vi "Client - Main.vi"() -> ()   [LabVIEW 2020]
uses:
  shared/controls/Ports to Check.ctl
  shared/controls/Client States.ctl
panel:
  out "Message from Server":string
  out "Connection Established?":bool
  in  "InsightCM Server Address":string="127.0.0.1"
  in  "User Panel":enum32{"User Panel"}(tab)
  in  "stop":bool
  in  "Establish Connection":bool
  in  "Start Test":bool
  in  "View Results":bool
  in  "Log Results":bool
  out "error out":errorcluster
  out "Ports to Check":T1={"TCP Ports"=[82, 482, 5672, 6343, 8002, 49580, 3580, 80, 22, 44516, 52725, 8080], "UDP Ports"=[5353, 44515, 44525]}
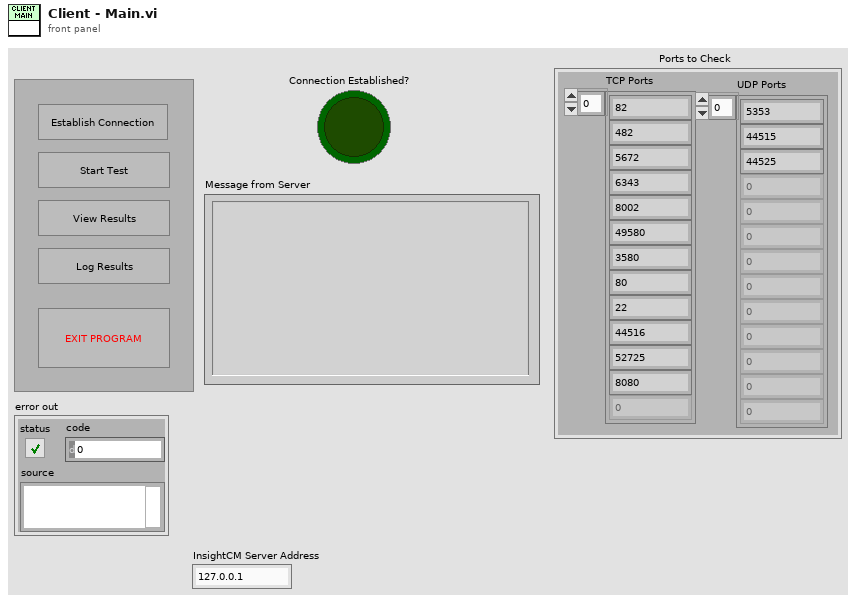
[diagram p1: front panel]
types:
  T1 = typedef "Ports to Check.ctl" = cluster{"TCP Ports":u32[], "UDP Ports":u32[]}
  T2 = typedef "Client States.ctl" = enum16{"Initialize", "Idle", "Establish Connection", "Start Test", "TCP Tests", "UDP Tests", "Test Complete", "View Results", "Log Results", "Edit Configuration", "Stop"}
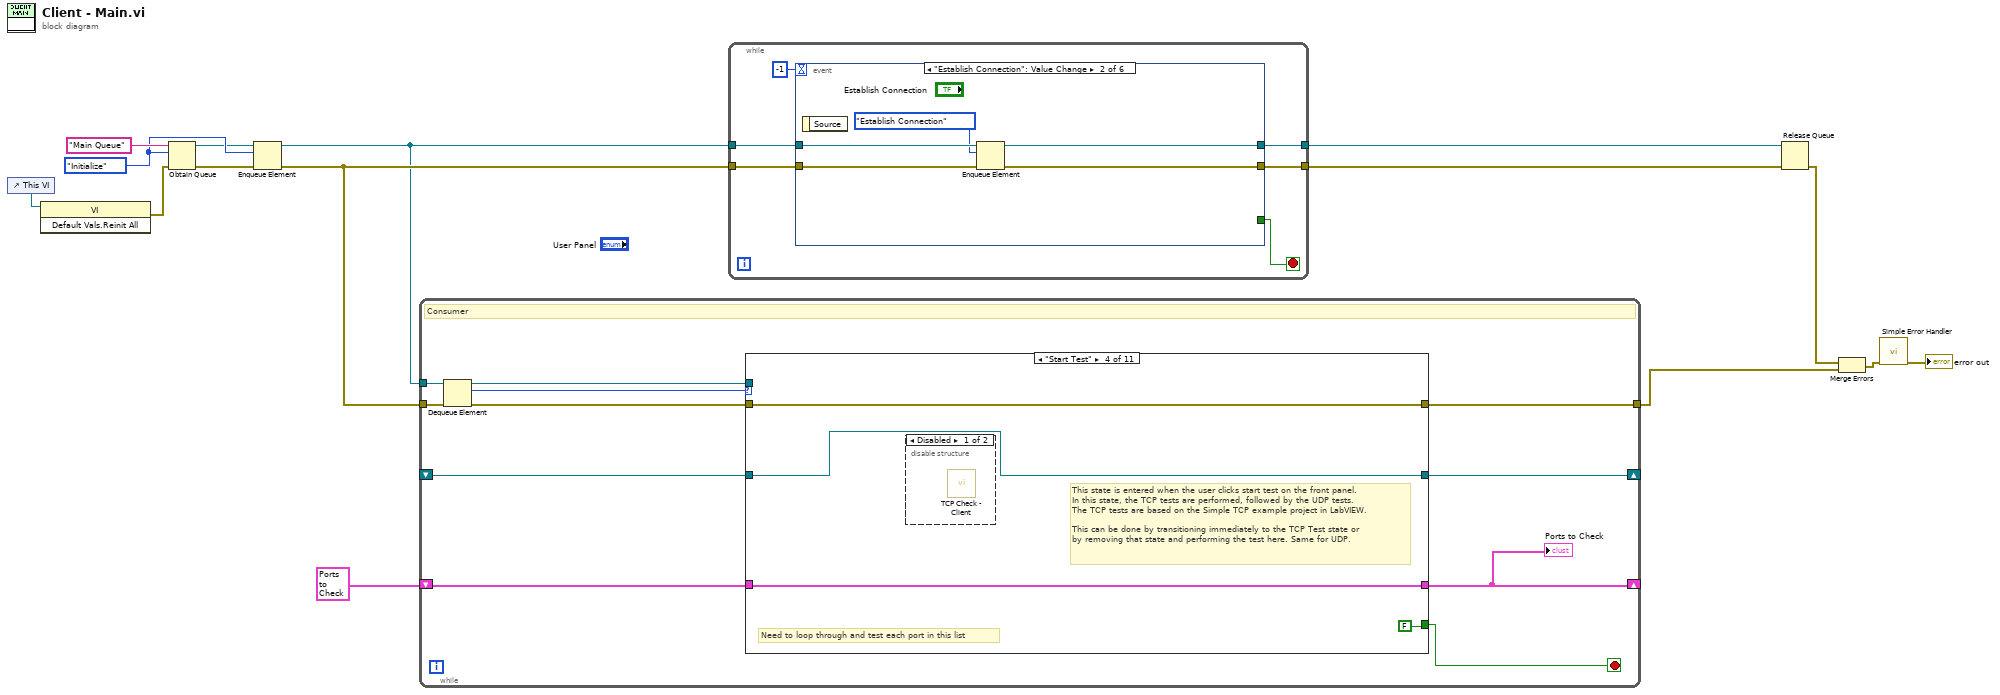
[diagram p0: block diagram]
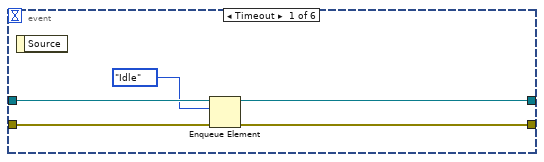
[diagram p2: hidden frame]
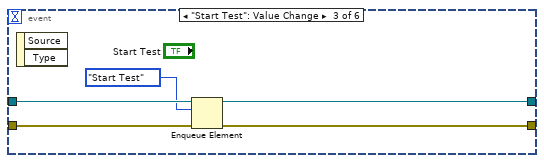
[diagram p3: hidden frame]
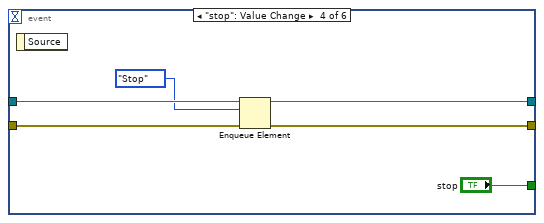
[diagram p4: hidden frame]
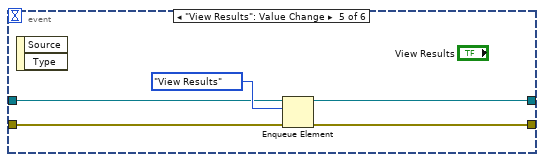
[diagram p5: hidden frame]
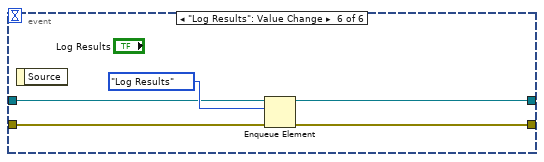
[diagram p6: hidden frame]
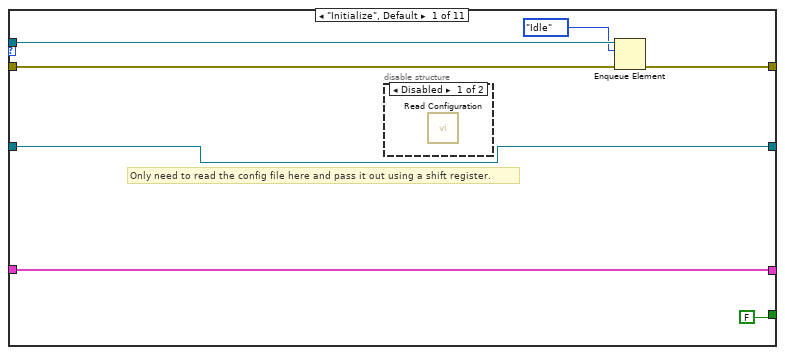
[diagram p7: hidden frame]
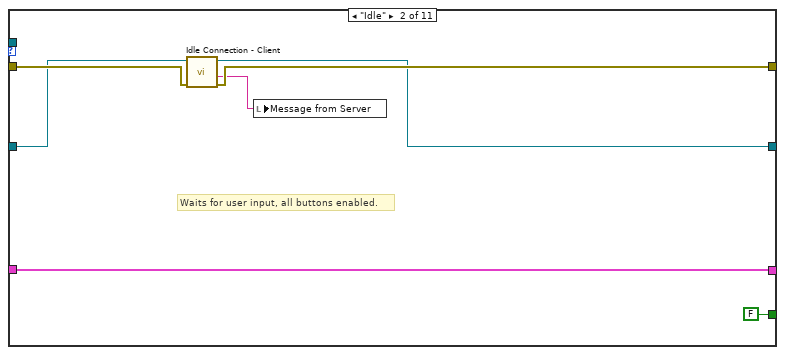
[diagram p9: hidden frame]
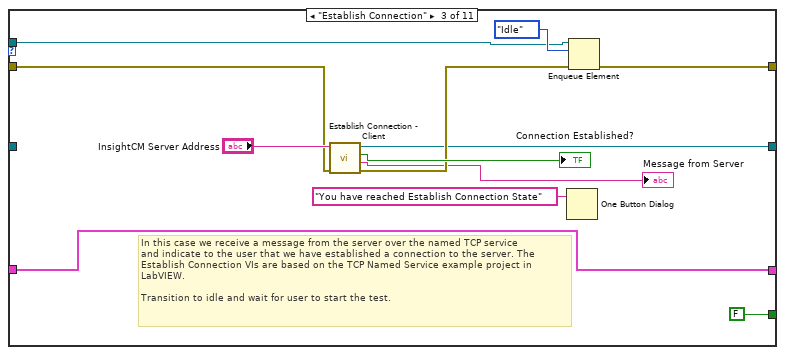
[diagram p10: hidden frame]
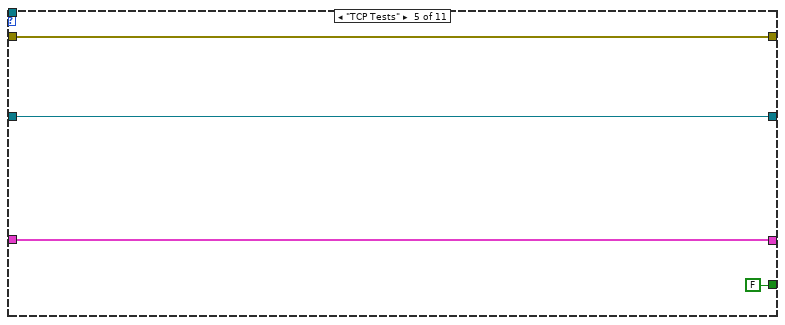
[diagram p12: hidden frame]
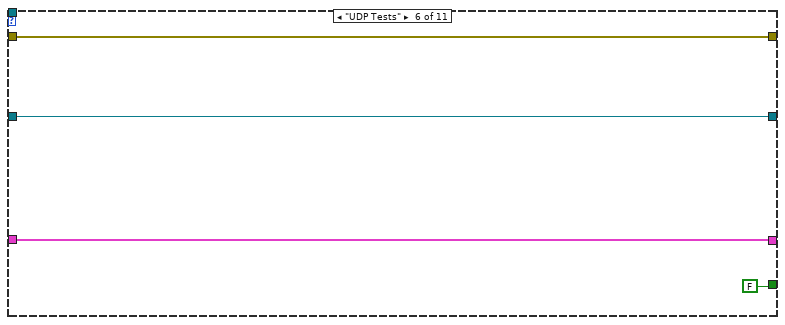
[diagram p13: hidden frame]
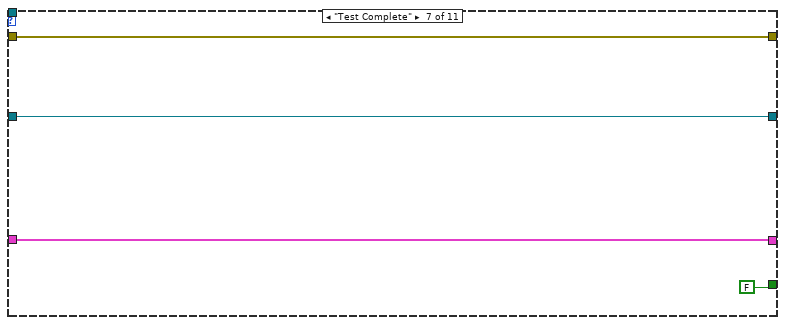
[diagram p14: hidden frame]
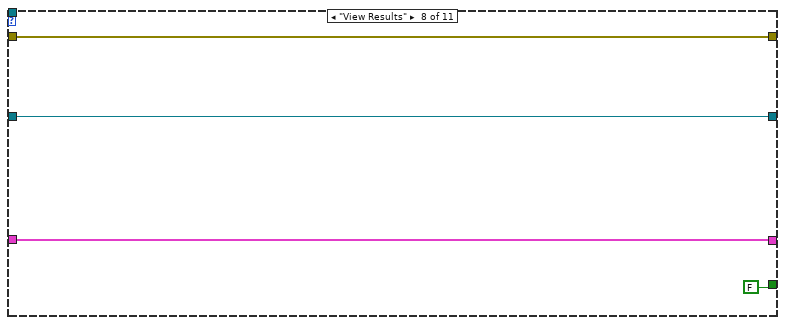
[diagram p15: hidden frame]
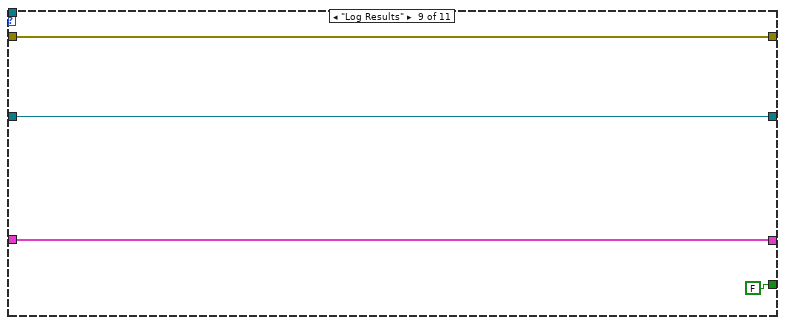
[diagram p16: hidden frame]
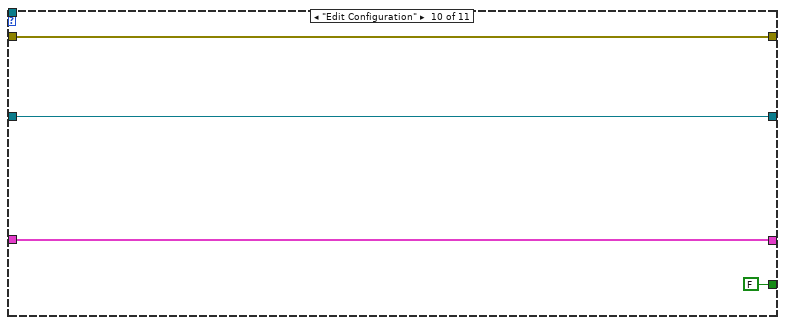
[diagram p17: hidden frame]
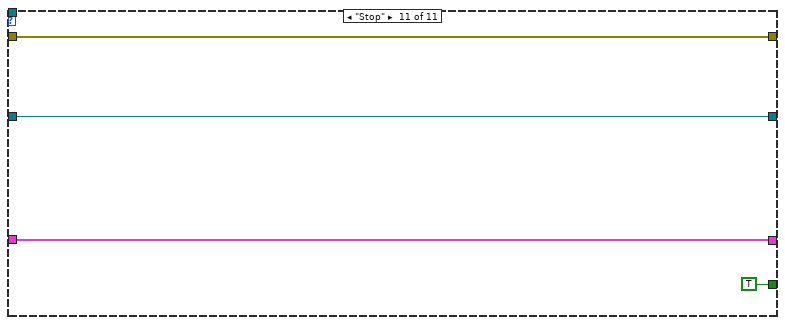
[diagram p18: hidden frame]
diagram:
  w5 = Client_States."Initialize" ("States")
  n1 = control-ref of="This VI"() -> (w8:refnum<vi>)
  n2 = invoke class="VI" method="Default Vals.Reinit All"(reference=w8) -> (error out=w7:errorcluster)  [unwired: 2 in, 2 out]
  n3 = Obtain Queue(name (unnamed)="Main Queue", element data type=w5, error in (no error)=w7) -> (queue out=w3:refnum<queue>, error out=w9:errorcluster)  [unwired: 2 in, 1 out]
  n4 = Enqueue Element(queue=w3, element=w5, error in (no error)=w9) -> (queue out=w4:refnum<queue>, error out=w6:errorcluster)  [unwired: 1 in, 1 out]
  n5 = while {
    tunnel: w4 -> [w26]
    tunnel: w6 -> [w25]
    shift-right: [w22] -> _
    shift-left: T1 {"TCP Ports"=[82, 482, 5672, 6343, 8002, 49580, 3580, 80, 22, 44516, 52725, 8080], "UDP Ports"=[5353, 44515, 44525]} ("Ports to Check") -> [w21]
    tunnel: [w19] -> w1
    shift-right: [w17] -> _
    shift-left: _ -> [w16]
    stop <- w18 stop-if-true
    # "Consumer"
    n6 = Dequeue Element(queue=w26, error in (no error)=w25) -> (queue out=w23:refnum<queue>, element=w24:T2, error out=w20:errorcluster)  [unwired: 1 in, 1 out]
    n7 = case shown="\"Start Test\"" w24 {
      tunnel: w23 -> [w33 _ w49 _ _ _ _ _ _ _ _]
      tunnel: [w30 w40 w51 w56 w60 w64 w68 w72 w76 w80 w84] -> w22
      tunnel: w21 -> [w30 w40 w51 w56 w60 w64 w68 w72 w76 w80 w84]
      tunnel: w20 -> [w31 w38 w46 w55 w59 w63 w67 w71 w75 w79 w83]
      tunnel: [w28 w36 w48 w55 w59 w63 w67 w71 w75 w79 w83] -> w19
      tunnel: [FALSE FALSE FALSE FALSE FALSE FALSE FALSE FALSE FALSE FALSE TRUE] -> w18
      tunnel: [w27 w35 w41 w53 w57 w61 w65 w69 w73 w77 w81] -> w17
      tunnel: w16 -> [w27 w37 _ w53 w57 w61 w65 w69 w73 w77 w81]
      frame "Initialize", Default {
        # "Only need to read the config file here and pass it out using a shift register."
        n8 = disable-structure shown="Disabled" {
          frame Disabled {
            n9 = call "Read Configuration.vi"() -> ()  [unwired: 10 in, 2 out]
          }
          frame Enabled {
          }
        }
        n10 = Enqueue Element(queue=w33, element=Client_States."Idle" ("States"), error in (no error)=w31) -> (error out=w28:errorcluster)  [unwired: 1 in, 2 out]
      }
      frame "Idle" {
        # "Waits for user input, all buttons enabled."
        n11 = call "Idle Connection - Client.vi"("connection ID"=w37, "error in (no error)"=w38) -> ("connection ID out"=w35:refnum<k5>, "Message from Server"=w34:string, "No error"=w36:errorcluster)  [unwired: 5 in, 1 out]
        n12 = local write "Message from Server"(w34) -> ()
      }
      frame "Establish Connection" {
        # "In this case we receive a message from the server over the named TCP service \nand indicate to the user that we have established a connection to the server. The \nEstablish Connection VIs are based on the TCP Named Service example project in \nLabVIEW. \n\nTransition to idle and wait for user to start the test."
        n13 = call "Establish Connection - Client.vi"("server address"="InsightCM Server Address", "error in (no error)"=w46) -> ("connection ID out"=w41:refnum<k5>, "Connection Established?"=→"Connection Established?":bool, "Message from Server"=→"Message from Server":string, "No error"=w45:errorcluster)  [unwired: 5 in]
        n14 = One Button Dialog(message="You have reached Establish Connection State") -> ()  [unwired: 1 in, 1 out]
        n15 = Enqueue Element(queue=w49, element=Client_States."Idle" ("States"), error in (no error)=w45) -> (error out=w48:errorcluster)  [unwired: 1 in, 2 out]
      }
      frame "Start Test" {
        # "Need to loop through and test each port in this list"
        # "This state is entered when the user clicks start test on the front panel.\nIn this state, the TCP tests are performed, followed by the UDP tests.\nThe TCP tests are based on the Simple TCP example project in LabVIEW.\n\nThis can be done by transitioning immediately to the TCP Test state or \nby removing that state and performing the test here. Same for UDP."
        n16 = disable-structure shown="Disabled" {
          frame Disabled {
            n17 = call "TCP Check - Client.vi"() -> ()  [unwired: 8 in, 3 out]
          }
          frame Enabled {
          }
        }
      }
      frame "TCP Tests" {
      }
      frame "UDP Tests" {
      }
      frame "Test Complete" {
      }
      frame "View Results" {
      }
      frame "Log Results" {
      }
      frame "Edit Configuration" {
      }
      frame "Stop" {
      }
    }
    "Ports to Check" <- w22
  }
  n18 = while {
    tunnel: w4 -> [w90]
    tunnel: [w89] -> w14
    tunnel: w6 -> [w87]
    tunnel: [w86] -> w11
    stop <- w88 stop-if-true
    n19 = event shown="[1] \"Establish Connection\": Value Change" {
      selector: _ -> [_ _ _ _ _ _]
      dyn-events: _ -> [_ _ _ _ _ _]
      timeout: -1 -> [_ _ _ _ _ _]
      tunnel: w90 -> [w95 w100 w105 w110 w115 w120]
      tunnel: [w94 w98 w103 w109 w114 w119] -> w89
      tunnel: [_ _ _ "stop" _ _] -> w88
      tunnel: w87 -> [w93 w97 w102 w107 w113 w118]
      tunnel: [w92 w96 w101 w106 w112 w117] -> w86
      event Timeout {
        n20 = event-data() -> ()  [unwired: 1 in, 1 out]
        n21 = Enqueue Element(queue=w95, element=Client_States."Idle" ("States"), error in (no error)=w93) -> (queue out=w94:refnum<queue>, error out=w92:errorcluster)  [unwired: 1 in, 1 out]
      }
      event "Establish Connection": Value Change {
        n22 = event-data() -> ()  [unwired: 1 in, 1 out]
        n23 = Enqueue Element(queue=w100, element=Client_States."Establish Connection" ("States"), error in (no error)=w97) -> (queue out=w98:refnum<queue>, error out=w96:errorcluster)  [unwired: 1 in, 1 out]
      }
      event "Start Test": Value Change {
        n24 = event-data() -> ()  [unwired: 1 in, 2 out]
        n25 = Enqueue Element(queue=w105, element=Client_States."Start Test" ("States"), error in (no error)=w102) -> (queue out=w103:refnum<queue>, error out=w101:errorcluster)  [unwired: 1 in, 1 out]
      }
      event "stop": Value Change {
        n26 = event-data() -> ()  [unwired: 1 in, 1 out]
        n27 = Enqueue Element(queue=w110, element=Client_States."Stop" ("States"), error in (no error)=w107) -> (queue out=w109:refnum<queue>, error out=w106:errorcluster)  [unwired: 1 in, 1 out]
      }
      event "View Results": Value Change {
        n28 = event-data() -> ()  [unwired: 1 in, 2 out]
        n29 = Enqueue Element(queue=w115, element=Client_States."View Results" ("States"), error in (no error)=w113) -> (queue out=w114:refnum<queue>, error out=w112:errorcluster)  [unwired: 1 in, 1 out]
      }
      event "Log Results": Value Change {
        n30 = event-data() -> ()  [unwired: 1 in, 1 out]
        n31 = Enqueue Element(queue=w120, element=Client_States."Log Results" ("States"), error in (no error)=w118) -> (queue out=w119:refnum<queue>, error out=w117:errorcluster)  [unwired: 1 in, 1 out]
      }
    }
  }
  n32 = Release Queue(queue=w14, error in (no error)=w11) -> (error out=w10:errorcluster)  [unwired: 1 in, 2 out]
  n33 = Merge Errors(w10, w1) -> (w12:errorcluster)
  n34 = call <vilib>:"Simple Error Handler.vi"("error in (no error)"=w12) -> ("error out"=→"error out":errorcluster)  [unwired: 4 in, 4 out]
